vi "PCO_SetModulationMode.vi"(5 "lMonitorOffset":i32, 6 "dwNumberOfExposures":u32, 7 "wTimebasePeriodical":u16(ring) items=["ns", "us", "ms"], 8 "error in (no error)":errorcluster {"code" format="%x"}, 9 "dwPeriodicalTime":u32, 10 "wModulationMode":u16(ring) items=["OFF", "ON"], 11 "ph":u64) -> (0 "error out":errorcluster {"code" format="%x"}, 2 "ErrorMessage":i32 format="%x", 3 "ph out":u64)   [LabVIEW 2019, in "SDK.lvlib" / "TimingControl.lvlib"]
doc: "<b>Description:</b>\nThis function does set the modulation mode and its corresponding parameters.\nThe modulation mode is an optional feature which is not available for all camera models. To determine if modulation mode is available first check if second descriptor is loadable through flag ENHANCED_DESCRIPTOR_2 in dwGeneralCapsDESC1 of PCO_Description structure. Then the presence of flag MODULATE in dwModulateCapsDESC2 of PCO_Description2 structure must be checked.\nRestrictions for the parameter values are defined through the timing values in the camera description PCO_Description2 structure.\n\n<b>Supported camera type:</b>\nAvailable for special versions of pco.1600, pco.2000 and pco.4000\n\n<b>Descriptor dependency:</b>\ndwGeneralCapsDESC1: ENHANCED_DESCRIPTOR_2\ndwModulateCapsDESC2: MODULATE"
uses:
  TimingControl.lvlib
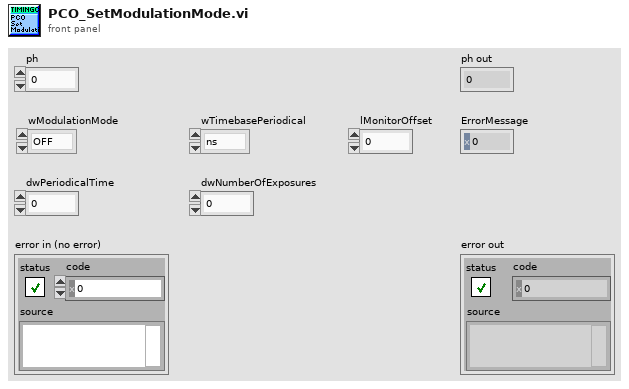
[diagram p1: front panel]
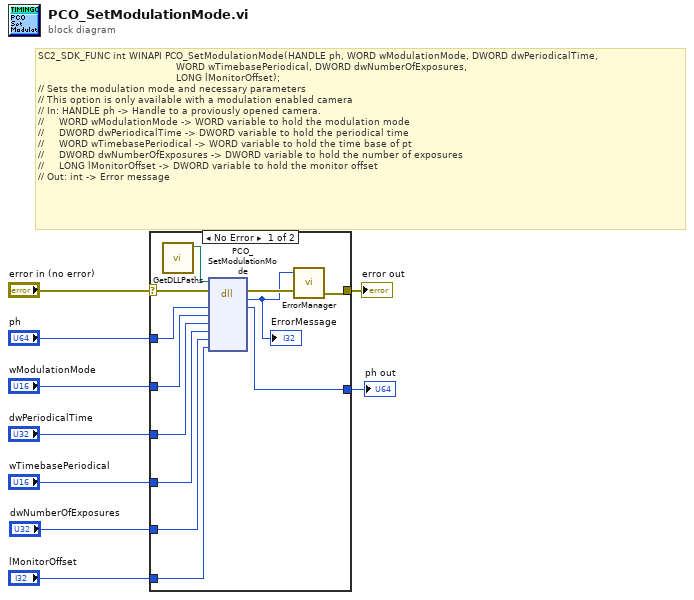
[diagram p0: block diagram]
diagram:
  # "SC2_SDK_FUNC int WINAPI PCO_SetModulationMode(HANDLE ph, WORD wModulationMode, DWORD dwPeriodicalTime,\n                                              WORD wTimebasePeriodical, DWORD dwNumberOfExposures,\n                                              LONG lMonitorOffset);\n// Sets the modulation mode and necessary parameters\n// This option is only available with a modulation enabled camera\n// In: HANDLE ph -> Handle to a proviously opened camera.\n//     WORD wModulationMode -> WORD variable to hold the modulation mode\n//     DWORD dwPeriodicalTime -> DWORD variable to hold the periodical time\n//     WORD wTimebasePeriodical -> WORD variable to hold the time base of pt\n//     DWORD dwNumberOfExposures -> DWORD variable to hold the number of exposures\n//     LONG lMonitorOffset -> DWORD variable to hold the monitor offset\n// Out: int -> Error message"
  n1 = case shown="No Error" "error in (no error)" {
    selector: "error in (no error)" -> [w14 w23]
    tunnel: "ph" -> [w21 w22]
    tunnel: [w20 w22] -> w8
    tunnel: "wModulationMode" -> [w19 _]
    tunnel: "dwPeriodicalTime" -> [w18 _]
    tunnel: "wTimebasePeriodical" -> [w17 _]
    tunnel: "dwNumberOfExposures" -> [w16 _]
    tunnel: "lMonitorOffset" -> [w15 _]
    tunnel: [w12 w23] -> w2
    frame No Error {
      n2 = call "GetDLLPaths.vi"() -> ("SC2_Cam_Path"=w10:path)  [unwired: 9 in, 2 out]
      n3 = dll-call lib="?" fn="PCO_SetModulationMode"(path in=w10, error in=w14, "ph"=w21, "wModulationMode"=w19, "dwPeriodicalTime"=w18, "wTimebasePeriodical"=w17, "dwNumberOfExposures"=w16, "lMonitorOffset"=w15) -> (error out=w13:errorcluster, "return type"=w11:i32, "ph"=w20:u64)  [unwired: 6 in, 1 out]
      "ErrorMessage" <- w11
      n4 = call "ErrorManager.vi"("error in (no error)"=w13, "error code"=w11) -> ("error out"=w12:errorcluster)  [unwired: 3 in]
    }
    frame Error {
    }
  }
  "ph out" <- w8
  "error out" <- w2
